vi "Begin.vi"(8 "error in":errorcluster) -> (0 "error out":errorcluster)   [LabVIEW 2018]
doc: "Called before other user functions, this VI is expected to open initial I/O refnums, load in file data, and do all program initialization. Notice that the <B>error out</B> terminal is simply used for data flow. Wiring it to other structures or subVIs ensures that this VI runs first."
uses:
  <vilib>/Rock Robotics/WPI/Joystick/WPI_JoystickDeviceEnum.ctl
  <vilib>/Rock Robotics/WPI/SafetyOutput/WPI_SafetyOutputConfigMenu.ctl
  <vilib>/Rock Robotics/WPI/DriverStation/WPI_DriverStationRobotMode2.ctl
  <vilib>/Rock Robotics/WPI/Solenoid/WPI_SolenoidChannel.ctl
  <vilib>/Rock Robotics/SystemInterfaces/DIO/FPGA_DIOPWMChannel.ctl
  <vilib>/Rock Robotics/WPI/ThirdParty/REV Robotics/SPARK MAX/Typedef/Spark MAX Idle Mode.ctl
  <vilib>/Rock Robotics/SystemInterfaces/DIO/FPGA_DIOChannel.ctl
  <vilib>/Rock Robotics/WPI/RobotDrive/WPI_RobotDriveOpen2MotorWithExistingMotors.vi
  Robot Global Data.vi
  <vilib>/Rock Robotics/WPI/Solenoid/WPI_SolenoidOpenDouble.vi
  <vilib>/Rock Robotics/WPI/MotorControl/WPI_MotorControlOpen VictorSP.vi
  <vilib>/Rock Robotics/WPI/Counter/WPI_CounterDigitalInputToDigitalSource.vi
  <vilib>/Rock Robotics/WPI/Switch/WPI_SwitchOpenLimit.vi
  <vilib>/Rock Robotics/WPI/Counter/WPI_CounterOpen UpDown Mode.vi
  <vilib>/Rock Robotics/WPI/Utilities/WPI_GetSetVariantRefNum.vi
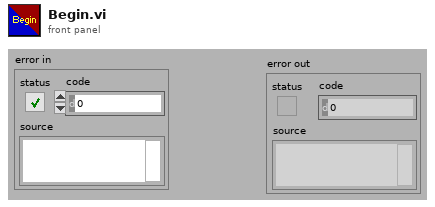
[diagram p1: front panel]
types:
  T1 = typedef "FPGA_DIOChannel.ctl" = enum8{"DIO 0", "DIO 1", "DIO 2", "DIO 3", "DIO 4", "DIO 5", "DIO 6", "DIO 7", "DIO 8", "DIO 9", "DIO MXP 0", "DIO MXP 1", "DIO MXP 2", "DIO MXP 3", "DIO MXP 4", "DIO MXP 5", "DIO MXP 6", "DIO MXP 7", "DIO MXP 8", "DIO MXP 9", "DIO MXP 10", "DIO MXP 11", "DIO MXP 12", "DIO MXP 13", "DIO MXP 14", "DIO MXP 15", "SPI Port CS1", "SPI Port CS2", "SPI Port CS3", "SPI Port MISO", "SPI Port MOSI", "Invalid"}
  T2 = typedef "FPGA_DIOPWMChannel.ctl" = enum8{"PWM 0", "PWM 1", "PWM 2", "PWM 3", "PWM 4", "PWM 5", "PWM 6", "PWM 7", "PWM 8", "PWM 9", "PWM MXP 0", "PWM MXP 1", "PWM MXP 2", "PWM MXP 3", "PWM MXP 4", "PWM MXP 5", "PWM MXP 6", "PWM MXP 7", "PWM MXP 8", "PWM MXP 9", "Invalid"}
  T3 = enum16{"Rising Edge", "Falling Edge", "Raising & Falling Edge", "Disabled"}
  T4 = typedef "WPI_JoystickDeviceEnum.ctl" = enum16{"USB 0", "USB 1", "USB 2", "USB 3", "USB 4", "USB 5"}
  T5 = typedef "Spark MAX Idle Mode.ctl" = enum16{"Coast", "Brake"}
  T6 = typedef "WPI_SolenoidChannel.ctl" = enum8{"Solenoid 0", "Solenoid 1", "Solenoid 2", "Solenoid 3", "Solenoid 4", "Solenoid 5", "Solenoid 6", "Solenoid 7", "Invalid"}
  T7 = typedef "WPI_DriverStationRobotMode2.ctl" = enum16{"Autonomous Disabled", "Autonomous Enabled", "Teleop Disabled", "Teleop Enabled", "Disconnected", "Finish", "Test Disabled", "Test Enabled", "Emergency Stopped"}
  T8 = typedef "WPI_SafetyOutputConfigMenu.ctl" = enum16{"Enable", "Disable"}
  T9 = typedef "WPI_CompressorDevRef.ctl" = cluster{"DevStatus":errorcluster, "Pneumatics Control Module":u8}
  T10 = typedef "WPI_MotorControlDeviceRef.ctl" = cluster{"DeviceStatus":errorcluster, "Type":T11, "PWM":cluster{"PWM Channel":T2, "DeadBand":T12}, "CAN":cluster{"Device Number":u8, "SetOutput VI Ref":variant, "GetOutput VI Ref":variant, "Enable VI Ref":variant, "Disable VI Ref":variant, "Data":variant}, "Invert":bool, "DIO PWM":cluster{"PWM \"Enable\" Channel":T2, "DIOChannel":T1, "PWM Rate":dbl}}
  T11 = typedef "WPI_MotorControlType.ctl" = enum16{"PWM", "CAN", "DIO PWM"}
  T12 = typedef "WPI_PWMDeadband.ctl" = cluster{"Name":string, "maxPositivePwm":i32, "minPositivePwm":i32, "centerPwm":i32, "maxNegativePwm":i32, "minNegativePwm":i32, "angularRange":u16}
  T13 = typedef "WPI_JoystickDevRef.ctl" = cluster{"Device":T4}
  T14 = typedef "WPI_DigitalInputDevRef.ctl" = cluster{"DevStatus":errorcluster, "DIO Channel":T1}
  T15 = typedef "FPGA_CounterEncoderSourceConvertionLVSourceType.ctl" = cluster{"DevStatus":errorcluster, "AnalogTriggerMode?":bool, "DigitalMode":cluster{"DIO Channel":T16}, "AnalogTriggerMode":cluster{"AnalogTriggerIndex":T17, "OutputType":T18}}
  T16 = typedef "FPGA_DIODigitalSourceChannel.ctl" = enum8{"DIO 0", "DIO 1", "DIO 2", "DIO 3", "DIO 4", "DIO 5", "DIO 6", "DIO 7", "DIO 8", "DIO 9", "DIO MXP 0", "DIO MXP 1", "DIO MXP 2", "DIO MXP 3", "DIO MXP 4", "DIO MXP 5", "DIO MXP 6", "DIO MXP 7", "DIO MXP 8", "DIO MXP 9", "DIO MXP 10", "DIO MXP 11", "DIO MXP 12", "DIO MXP 13", "DIO MXP 14", "DIO MXP 15", "SPI Port CS1", "SPI Port CS2", "SPI Port CS3", "SPI Port MISO", "SPI Port MOSI", "Disabled"}
  T17 = typedef "FPGA_AnalogTriggerIndex.ctl" = enum8{"Trig 0", "Trig 1", "Trig 2", "Trig 3", "Trig 4", "Trig 5", "Trig 6", "Trig 7", "Invalid"}
  T18 = typedef "FPGA_AnalogTriggerOutType.ctl" = enum16{"InWindow", "TriggerState", "Rising", "Falling"}
  T19 = typedef "WPI_RobotDriveDevRef.ctl" = cluster{"DevStatus":errorcluster, "Motors[]":T10[], "Square Inputs":bool, "Max Output":dbl}
  T20 = typedef "WPI_CounterDevRef.ctl" = cluster{"DevStatus":errorcluster, "CntIndex":T21}
  T21 = typedef "FPGA_CounterCtrSystemIndex.ctl" = enum8{"Ctr 0", "Ctr 1", "Ctr 2", "Ctr 3", "Ctr 4", "Ctr 5", "Ctr 6", "Ctr 7", "Invalid"}
  T22 = typedef "WPI_EncoderDevRef.ctl" = cluster{"DevStatus":errorcluster, "EncoderIndex":T23, "CounterIndex":T21, "DistancePerCount":dbl, "Decoding Type":T24}
  T23 = typedef "FPGA_EncoderIdx.ctl" = enum8{"Enc 0", "Enc 1", "Enc 2", "Enc 3", "Enc 4", "Enc 5", "Enc 6", "Enc 7", "Invalid"}
  T24 = typedef "WPI_EncoderType.ctl" = enum16{"1x", "2x", "4x"}
  T25 = typedef "WPI_SolenoidDevRef.ctl" = cluster{"DevStatus":errorcluster, "Pneumatics Control Module":u8, "Forward Solenoid Channel":T6, "Reverse Solenoid Channel":T6}
  T26 = typedef "WPI_SwitchDevRef.ctl" = cluster{"DevStatus":errorcluster, "DIO Channel":T1, "CntIndex":T21, "Normally Closed":bool}
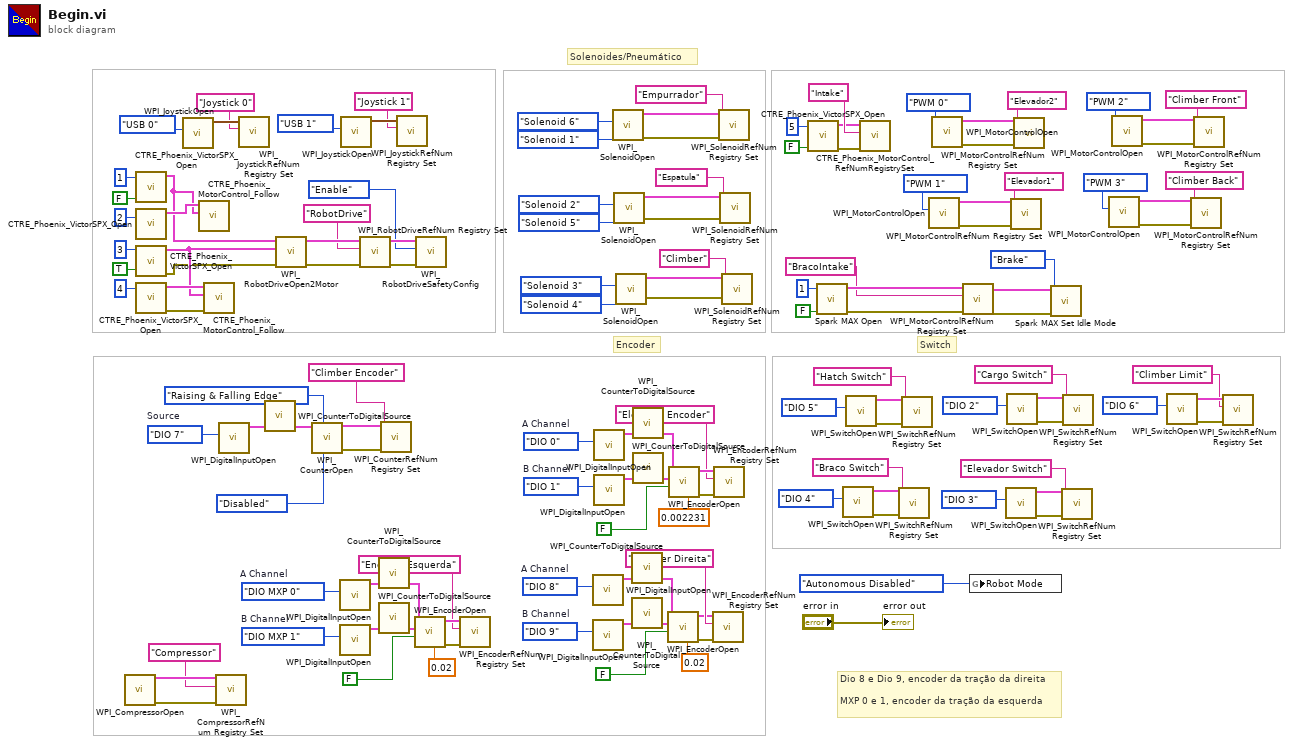
[diagram p0: block diagram]
diagram:
  w14 = FPGA_DIOChannel."DIO MXP 1"  # B Channel
  w13 = FPGA_DIOChannel."DIO MXP 0"  # A Channel
  w15 = FPGA_DIOChannel."DIO 9"  # B Channel
  w16 = FPGA_DIOChannel."DIO 8"  # A Channel
  w44 = FPGA_DIOChannel."DIO 7"  # Source
  w75 = FPGA_DIOChannel."DIO 1"  # B Channel
  w74 = FPGA_DIOChannel."DIO 0"  # A Channel
  # "Dio 8 e Dio 9, encoder da tração da direita\n\nMXP 0 e 1, encoder da tração da esquerda"
  # "Encoder"
  # "Switch"
  # "Solenoides/Pneumático"
  n1 = call <vilib>:"WPI_CompressorOpen.vi"() -> ("CompressorDevRef"=w3:T9, "error out"=w2:errorcluster)  [unwired: 14 in]
  n2 = call <vilib>:"CTRE_Phoenix_VictorSPX_Open.vi"("Invert"=FALSE, "Device Number"=u8 1) -> ("CAN Talon SRX Ref"=w113:T10)  [unwired: 8 in, 1 out]
  n3 = call <vilib>:"CTRE_Phoenix_VictorSPX_Open.vi"("Device Number"=u8 2) -> ("CAN Talon SRX Ref"=w114:T10)  [unwired: 9 in, 1 out]
  n4 = call <vilib>:"CTRE_Phoenix_VictorSPX_Open.vi"("Invert"=TRUE, "Device Number"=u8 3) -> ("error out"=w121:errorcluster, "CAN Talon SRX Ref"=w129:T10)  [unwired: 8 in]
  n5 = call <vilib>:"CTRE_Phoenix_VictorSPX_Open.vi"("Device Number"=u8 4) -> ("error out"=w122:errorcluster, "CAN Talon SRX Ref"=w130:T10)  [unwired: 9 in]
  n6 = call <vilib>:"WPI_JoystickOpen.vi"("JoystickDevice"=WPI_JoystickDeviceEnum."USB 0") -> ("JoystickDevRef"=w133:T13)  [unwired: 10 in]
  n7 = call <vilib>:"CTRE_Phoenix_MotorControl_Follow.vi"("Master Controller to Follow"=w113, "PhoenixMotorControlDevRef"=w114) -> ()  [unwired: 8 in, 2 out]
  n8 = call <vilib>:"CTRE_Phoenix_MotorControl_Follow.vi"("error in (no error)"=w122, "Master Controller to Follow"=w129, "PhoenixMotorControlDevRef"=w130) -> ()  [unwired: 7 in, 2 out]
  n9 = call <vilib>:"WPI_CompressorRefNum Registry Set.vi"("error in (no error)"=w2, "refnum name"="Compressor", "CompressorDevRef"=w3) -> ()  [unwired: 7 in, 2 out]
  n10 = call <vilib>:"WPI_DigitalInputOpen.vi"("DIO Channel"=w44) -> ("DigitalInputDevRef"=w43:T14)  [unwired: 1 in, 9 out]
  n11 = call <vilib>:"WPI_JoystickRefNum Registry Set.vi"("refnum name"="Joystick 0", "JoystickDevRef"=w133) -> ()  [unwired: 8 in, 2 out]
  n12 = call-poly <vilib>:"WPI_CounterToDigitalSource.vi"("DigitalInputDevRef"=w43) -> ("Digital Source"=w45:T15)  [unwired: 6 out]
  n13 = call-poly <vilib>:"WPI_RobotDriveOpen2Motor.vi"("error in (no error)"=w121, "Right Motor Dev Ref"=w129, "Left Motor Dev Ref"=w113) -> ("error out"=w120:errorcluster, "RobotDriveDevRef"=w119:T19)  [unwired: 7 in]
  n14 = call-poly <vilib>:"WPI_CounterOpen.vi"("DownEdge"=T3."Disabled", "UpEdge"=T3."Raising & Falling Edge", "Up Source"=w45) -> ("error out"=w39:errorcluster, "CounterDevRef"=w40:T20)  [unwired: 4 in, 3 out]
  n15 = call <vilib>:"WPI_DigitalInputOpen.vi"("DIO Channel"=w13) -> ("DigitalInputDevRef"=w10:T14)  [unwired: 1 in, 9 out]
  n16 = call <vilib>:"WPI_DigitalInputOpen.vi"("DIO Channel"=w14) -> ("DigitalInputDevRef"=w11:T14)  [unwired: 1 in, 9 out]
  n17 = call <vilib>:"WPI_JoystickOpen.vi"("JoystickDevice"=WPI_JoystickDeviceEnum."USB 1") -> ("JoystickDevRef"=w50:T13)  [unwired: 10 in]
  n18 = call <vilib>:"WPI_RobotDriveRefNum Registry Set.vi"("error in (no error)"=w120, "refnum name"="RobotDrive", "RobotDriveDevRef"=w119) -> ("error out"=w117:errorcluster, "RobotDriveDevRef"=w116:T19)  [unwired: 7 in]
  n19 = call-poly <vilib>:"WPI_CounterToDigitalSource.vi"("DigitalInputDevRef"=w10) -> ("Digital Source"=w9:T15)  [unwired: 6 out]
  n20 = call-poly <vilib>:"WPI_CounterToDigitalSource.vi"("DigitalInputDevRef"=w11) -> ("Digital Source"=w12:T15)  [unwired: 6 out]
  n21 = call <vilib>:"WPI_CounterRefNum Registry Set.vi"("error in (no error)"=w39, "refnum name"="Climber Encoder", "CounterDevRef"=w40) -> ()  [unwired: 7 in, 2 out]
  n22 = call <vilib>:"WPI_JoystickRefNum Registry Set.vi"("refnum name"="Joystick 1", "JoystickDevRef"=w50) -> ()  [unwired: 8 in, 2 out]
  n23 = call <vilib>:"WPI_EncoderOpen.vi"("DistancePerCount"=0.02, "Invert Direction (False)"=FALSE, "BSource"=w12, "ASource"=w9) -> ("error out"=w8:errorcluster, "EncoderDevRef"=w7:T22)  [unwired: 4 in, 2 out]
  n24 = call <vilib>:"WPI_RobotDriveSafetyConfig.vi"("error in (no error)"=w117, "mode"=WPI_SafetyOutputConfigMenu."Enable", "RobotDriveDevRef"=w116) -> ()  [unwired: 7 in, 2 out]
  n25 = call <vilib>:"WPI_EncoderRefNum Registry Set.vi"("error in (no error)"=w8, "refnum name"="Encoder Esquerda", "EncoderDevRef"=w7) -> ()  [unwired: 7 in, 2 out]
  n26 = call <vilib>:"WPI_DigitalInputOpen.vi"("DIO Channel"=w16) -> ("DigitalInputDevRef"=w19:T14)  [unwired: 1 in, 9 out]
  n27 = call <vilib>:"WPI_DigitalInputOpen.vi"("DIO Channel"=w15) -> ("DigitalInputDevRef"=w18:T14)  [unwired: 1 in, 9 out]
  n28 = call <vilib>:"WPI_DigitalInputOpen.vi"("DIO Channel"=w74) -> ("DigitalInputDevRef"=w71:T14)  [unwired: 1 in, 9 out]
  n29 = call <vilib>:"WPI_DigitalInputOpen.vi"("DIO Channel"=w75) -> ("DigitalInputDevRef"=w72:T14)  [unwired: 1 in, 9 out]
  n30 = call-poly <vilib>:"WPI_SolenoidOpen.vi"("Reverse Solenoid Channel"=WPI_SolenoidChannel."Solenoid 1", "Forward Solenoid Channel"=WPI_SolenoidChannel."Solenoid 6") -> ("error out"=w108:errorcluster, "SolenoidDevRef"=w109:T25)  [unwired: 8 in]
  n31 = call-poly <vilib>:"WPI_SolenoidOpen.vi"("Reverse Solenoid Channel"=WPI_SolenoidChannel."Solenoid 5", "Forward Solenoid Channel"=WPI_SolenoidChannel."Solenoid 2") -> ("error out"=w105:errorcluster, "SolenoidDevRef"=w104:T25)  [unwired: 8 in]
  n32 = call-poly <vilib>:"WPI_SolenoidOpen.vi"("Reverse Solenoid Channel"=WPI_SolenoidChannel."Solenoid 4", "Forward Solenoid Channel"=WPI_SolenoidChannel."Solenoid 3") -> ("error out"=w100:errorcluster, "SolenoidDevRef"=w99:T25)  [unwired: 8 in]
  n33 = call-poly <vilib>:"WPI_CounterToDigitalSource.vi"("DigitalInputDevRef"=w19) -> ("Digital Source"=w20:T15)  [unwired: 6 out]
  n34 = call-poly <vilib>:"WPI_CounterToDigitalSource.vi"("DigitalInputDevRef"=w18) -> ("Digital Source"=w17:T15)  [unwired: 6 out]
  n35 = call-poly <vilib>:"WPI_CounterToDigitalSource.vi"("DigitalInputDevRef"=w71) -> ("Digital Source"=w70:T15)  [unwired: 6 out]
  n36 = call-poly <vilib>:"WPI_CounterToDigitalSource.vi"("DigitalInputDevRef"=w72) -> ("Digital Source"=w73:T15)  [unwired: 6 out]
  n37 = call <vilib>:"WPI_EncoderOpen.vi"("DistancePerCount"=0.02, "Invert Direction (False)"=FALSE, "BSource"=w17, "ASource"=w20) -> ("error out"=w21:errorcluster, "EncoderDevRef"=w22:T22)  [unwired: 4 in, 2 out]
  n38 = call <vilib>:"WPI_EncoderOpen.vi"("DistancePerCount"=0.002231, "Invert Direction (False)"=FALSE, "BSource"=w73, "ASource"=w70) -> ("error out"=w53:errorcluster, "EncoderDevRef"=w52:T22)  [unwired: 4 in, 2 out]
  n39 = call <vilib>:"WPI_EncoderRefNum Registry Set.vi"("error in (no error)"=w21, "refnum name"="Encoder Direita", "EncoderDevRef"=w22) -> ()  [unwired: 7 in, 2 out]
  n40 = call <vilib>:"WPI_EncoderRefNum Registry Set.vi"("error in (no error)"=w53, "refnum name"="Elevador Encoder", "EncoderDevRef"=w52) -> ()  [unwired: 7 in, 2 out]
  n41 = call <vilib>:"WPI_SolenoidRefNum Registry Set.vi"("error in (no error)"=w108, "refnum name"="Empurrador", "SolenoidDevRef"=w109) -> ()  [unwired: 7 in, 2 out]
  n42 = call <vilib>:"WPI_SolenoidRefNum Registry Set.vi"("error in (no error)"=w105, "refnum name"="Espatula", "SolenoidDevRef"=w104) -> ()  [unwired: 7 in, 2 out]
  n43 = call <vilib>:"WPI_SolenoidRefNum Registry Set.vi"("error in (no error)"=w100, "refnum name"="Climber", "SolenoidDevRef"=w99) -> ()  [unwired: 7 in, 2 out]
  n44 = call <vilib>:"CTRE_Phoenix_VictorSPX_Open.vi"("Invert"=FALSE, "Device Number"=u8 5) -> ("error out"=w94:errorcluster, "CAN Talon SRX Ref"=w92:T10)  [unwired: 8 in]
  n45 = call <vilib>:"Spark MAX Open.vi"("Invert"=FALSE, "Device Number"=u8 1) -> ("error out"=w83:errorcluster, "MotorControlDeviceRef"=w82:T10)  [unwired: 8 in]
  n46 = call-poly <vilib>:"WPI_SwitchOpen.vi"("DIO Channel"=FPGA_DIOChannel."DIO 4") -> ("error out"=w61:errorcluster, "SwitchDevRef"=w60:T26)  [unwired: 9 in]
  n47 = call-poly <vilib>:"WPI_SwitchOpen.vi"("DIO Channel"=FPGA_DIOChannel."DIO 5") -> ("error out"=w69:errorcluster, "SwitchDevRef"=w68:T26)  [unwired: 9 in]
  n48 = call <vilib>:"CTRE_Phoenix_MotorControl_RefNumRegistrySet.vi"("error in (no error)"=w94, "refnum name"="Intake", "PhoenixMotorControlDevRef"=w92) -> ()  [unwired: 7 in, 2 out]
  n49 = call <vilib>:"WPI_SwitchRefNum Registry Set.vi"("error in (no error)"=w61, "refnum name"="Braco Switch", "SwitchDevRef"=w60) -> ()  [unwired: 7 in, 2 out]
  n50 = call <vilib>:"WPI_SwitchRefNum Registry Set.vi"("error in (no error)"=w69, "refnum name"="Hatch Switch", "SwitchDevRef"=w68) -> ()  [unwired: 7 in, 2 out]
  n51 = call-poly <vilib>:"WPI_MotorControlOpen.vi"("PWM Channel"=FPGA_DIOPWMChannel."PWM 1") -> ("error out"=w86:errorcluster, "MotorControlDeviceRef"=w87:T10)  [unwired: 9 in]
  n52 = call-poly <vilib>:"WPI_MotorControlOpen.vi"("PWM Channel"=FPGA_DIOPWMChannel."PWM 0") -> ("error out"=w90:errorcluster, "MotorControlDeviceRef"=w91:T10)  [unwired: 9 in]
  n53 = call <vilib>:"WPI_MotorControlRefNum Registry Set.vi"("error in (no error)"=w83, "refnum name"="BracoIntake", "MotorControlDevRef"=w82) -> ("error out"=w77:errorcluster, "MotorControlDevRef"=w78:T10)  [unwired: 7 in]
  n54 = global write "Robot Global Data.vi" "Robot Mode"(WPI_DriverStationRobotMode2."Autonomous Disabled" ("Robot Mode")) -> ()
  n55 = call-poly <vilib>:"WPI_SwitchOpen.vi"("DIO Channel"=FPGA_DIOChannel."DIO 3") -> ("error out"=w57:errorcluster, "SwitchDevRef"=w56:T26)  [unwired: 9 in]
  n56 = call-poly <vilib>:"WPI_SwitchOpen.vi"("DIO Channel"=FPGA_DIOChannel."DIO 2") -> ("error out"=w65:errorcluster, "SwitchDevRef"=w64:T26)  [unwired: 9 in]
  n57 = call <vilib>:"WPI_MotorControlRefNum Registry Set.vi"("error in (no error)"=w86, "refnum name"="Elevador1", "MotorControlDevRef"=w87) -> ()  [unwired: 7 in, 2 out]
  n58 = call <vilib>:"WPI_MotorControlRefNum Registry Set.vi"("error in (no error)"=w90, "refnum name"="Elevador2", "MotorControlDevRef"=w91) -> ()  [unwired: 7 in, 2 out]
  n59 = call <vilib>:"Spark MAX Set Idle Mode.vi"("error in (no error)"=w77, "Idle Mode"=Spark_MAX_Idle_Mode."Brake", "MotorControlDeviceRef in"=w78) -> ()  [unwired: 7 in, 2 out]
  n60 = call <vilib>:"WPI_SwitchRefNum Registry Set.vi"("error in (no error)"=w57, "refnum name"="Elevador Switch", "SwitchDevRef"=w56) -> ()  [unwired: 7 in, 2 out]
  n61 = call <vilib>:"WPI_SwitchRefNum Registry Set.vi"("error in (no error)"=w65, "refnum name"="Cargo Switch", "SwitchDevRef"=w64) -> ()  [unwired: 7 in, 2 out]
  n62 = call-poly <vilib>:"WPI_MotorControlOpen.vi"("PWM Channel"=FPGA_DIOPWMChannel."PWM 3") -> ("error out"=w31:errorcluster, "MotorControlDeviceRef"=w30:T10)  [unwired: 9 in]
  n63 = call-poly <vilib>:"WPI_MotorControlOpen.vi"("PWM Channel"=FPGA_DIOPWMChannel."PWM 2") -> ("error out"=w27:errorcluster, "MotorControlDeviceRef"=w26:T10)  [unwired: 9 in]
  n64 = call-poly <vilib>:"WPI_SwitchOpen.vi"("DIO Channel"=FPGA_DIOChannel."DIO 6") -> ("error out"=w35:errorcluster, "SwitchDevRef"=w36:T26)  [unwired: 9 in]
  n65 = call <vilib>:"WPI_MotorControlRefNum Registry Set.vi"("error in (no error)"=w31, "refnum name"="Climber Back", "MotorControlDevRef"=w30) -> ()  [unwired: 7 in, 2 out]
  n66 = call <vilib>:"WPI_MotorControlRefNum Registry Set.vi"("error in (no error)"=w27, "refnum name"="Climber Front", "MotorControlDevRef"=w26) -> ()  [unwired: 7 in, 2 out]
  n67 = call <vilib>:"WPI_SwitchRefNum Registry Set.vi"("error in (no error)"=w35, "refnum name"="Climber Limit", "SwitchDevRef"=w36) -> ()  [unwired: 7 in, 2 out]
  "error out" <- "error in"
